vi "Build.vi"(8 "error in (no error)":errorcluster, 11 "Build in":refnum<class "AB_DepPackedLibrary.lvclass">) -> (0 "error out":errorcluster, 1 "GeneratedFiles":path[](array[path]), 2 "GeneratedDirectories":path[](array[path]), 3 "Build out":refnum<class "AB_DepPackedLibrary.lvclass">, 4 "GeneratedFileGUIDs":string[](array[string]), 5 "OutputDirectory":path, 7 "Dependencies":T1[](array[typedef]))   [LabVIEW 2020, in "AB_DepPackedLibrary.lvclass"]
uses:
  <vilib>/AppBuilder/AB_Classes/DepPackedLib/AB_DepPackedLibrary.lvclass
  <vilib>/AppBuilder/AB_Classes/DepPackedLib/AB_DepPackedLibrary.lvclass/AB_DepPackedLibrary.ctl
  <vilib>/AppBuilder/AB_Classes/Deployment/AB_Deployment.lvlib
  <vilib>/AppBuilder/AB_Classes/PackedLib/AB_PackedLibrary.lvclass
  e:/builds/penguin/labview/branches/2020/dev/dist/vi.lib/AppBuilder/AB_Classes/PackedLib/AB_PackedLibrary.lvclass
  e:/builds/penguin/labview/branches/2020/dev/dist/vi.lib/AppBuilder/AB_Classes/TargetFile/AB_Targetfile.lvclass
  e:/builds/penguin/labview/branches/2020/dev/dist/vi.lib/AppBuilder/AB_Classes/Build/AB_Build.lvclass
  e:/builds/penguin/labview/branches/2020/dev/dist/vi.lib/AppBuilder/AB_Classes/DepPackedLib/AB_DepPackedLibrary.lvclass
  <vilib>/Utility/lvfile.llb/LVFileType.ctl
  <vilib>/Utility/lvfile.llb/NI_FileType.lvlib
  <vilib>/AppBuilder/AB_Dependency.ctl
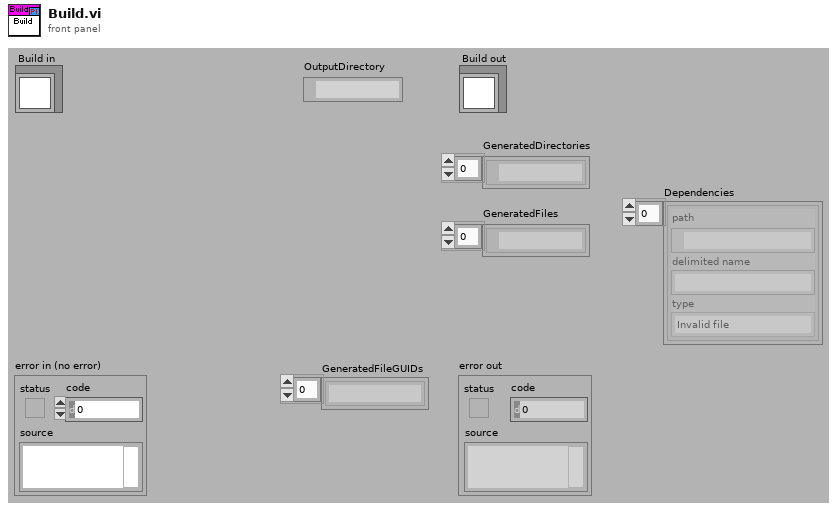
[diagram p1: front panel]
types:
  T1 = typedef "AB_Dependency.ctl" = cluster{"path":path, "delimited name":string, "type":T2}
  T2 = typedef "NI_FileType.lvlib/LVFileType.ctl" = enum32{"Invalid file", "Unknown type", "Instrument", "Control", "Polymorphic VI", "Project", "Library", "LVClass", "XControl", "XNode", "Shared library", ".NET assembly", "ActiveX interface", "CIN", "Run-time menu", "Palette menu", "Help file", "LLB", "XNode Edit Dependency", "Class Private Data Control", "Statechart", "MathScript .m file", "Ladder Diagram", "LVLibp", "XNode Build Dependency"}
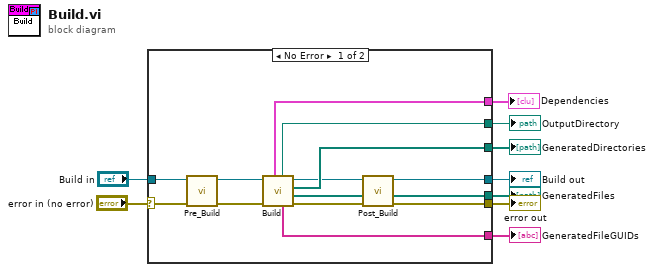
[diagram p0: block diagram]
diagram:
  n1 = case shown="No Error" "error in (no error)" {
    selector: "error in (no error)" -> [w17 w24]
    tunnel: [w21 _] -> w9
    tunnel: [w14 w25] -> w8
    tunnel: [w23 _] -> w7
    tunnel: [w22 _] -> w6
    tunnel: "Build in" -> [w19 w25]
    tunnel: [w12 w24] -> w4
    tunnel: [w11 _] -> w3
    tunnel: [w20 _] -> w1
    frame No Error {
      n2 = call <vilib>:"Pre_Build.vi"("error in (no error)"=w17, "Build in"=w19) -> ("error out"=w16:errorcluster, "Build out"=w18:refnum<class "AB_DepPackedLibrary.lvclass">)  [unwired: 8 in]
      n3 = call-parent "Build.vi"("error in (no error)"=w16, "Build in"=w18) -> ("error out"=w13:errorcluster, "GeneratedFiles"=w10:path[], "GeneratedDirectories"=w21:path[], "Build out"=w15:refnum<class "AB_DepPackedLibrary.lvclass">, "GeneratedFileGUIDs"=w23:string[], "OutputDirectory"=w22:path, "Dependencies"=w20:T1[])  [unwired: 3 in]
      n4 = call <vilib>:"Post_Build.vi"("error in (no error)"=w13, "generated files"=w10, "Build in"=w15) -> ("error out"=w12:errorcluster, "GeneratedFiles"=w11:path[], "Build out"=w14:refnum<class "AB_DepPackedLibrary.lvclass">)  [unwired: 6 in]
    }
    frame Error {
    }
  }
  "error out" <- w4
  "GeneratedFiles" <- w3
  "GeneratedDirectories" <- w9
  "Build out" <- w8
  "OutputDirectory" <- w6
  "GeneratedFileGUIDs" <- w7
  "Dependencies" <- w1
